vi "Connect Channel.vi"(7 "Channel Array in":refnum<class "CIFChannels.lvclass">[](array[class]), 8 "error in (no error)":errorcluster, 9 "Connection":T1 {"Custom Data" format="%.0x"}, 10 "Subscriber Name":string, 11 "CIFChannelMng in":refnum<class "CIFChannelMng.lvclass">) -> (0 "error out":errorcluster, 2 "Update OOB":bool, 3 "CIFChannelMng out":refnum<class "CIFChannelMng.lvclass">, 5 "Channel Array out":refnum<class "CIFChannels.lvclass">[](array[class]))   [LabVIEW 2021, in "CIFChannelMng.lvclass"]
uses:
  CIFChannelMng.lvclass
  CIFChannelMng.lvclass/CIFChannelMng.ctl
  <vilib>/CIF Foundation/CIF Channels Core/CIFChannels/Typedef/Channel State.ctl
  <vilib>/CIF Foundation/CIF Channels Core/CIFChannels/CIFChannels.lvclass
  <vilib>/CIF Foundation/CIF Channels Core/ChannelCommon/typedef/New FIFO Instance Response.ctl
  <vilib>/CIF Foundation/CIF Channels Core/ChannelCommon/ChannelCommon.lvlib
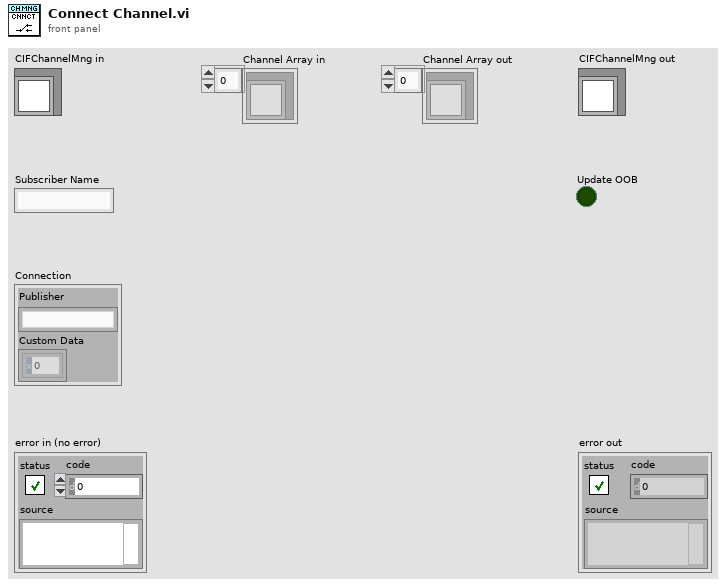
[diagram p1: front panel]
types:
  T1 = typedef "ChannelCommon.lvlib/New FIFO Instance Response.ctl" = cluster{"Publisher":string, "Custom Data":u8[]}
  T2 = typedef "CIFChannels.lvclass/Channel State.ctl" = enum16{"Creating", "Disconnected", "Connecting", "Connected", "Destroyed"}
  T3 = typedef "CIFChannelMng.lvclass/Channel List for OOB.ctl" = cluster{"Name":string, "Direction":T4, "Type":string, "Connected?":bool, "Connected Name":string, "Custom Config Data":u8[], "Forced?":bool, "Pattern":T5}
  T4 = typedef "CIFChannels.lvclass/Direction.ctl" = enum16{"Publisher", "Subscriber"}
  T5 = typedef "ChannelCommon.lvlib/Channel Pattern.ctl" = enum16{"Unknown", "Tag", "FIFO", "MultiFIFO", "BackpressureFIFO"}
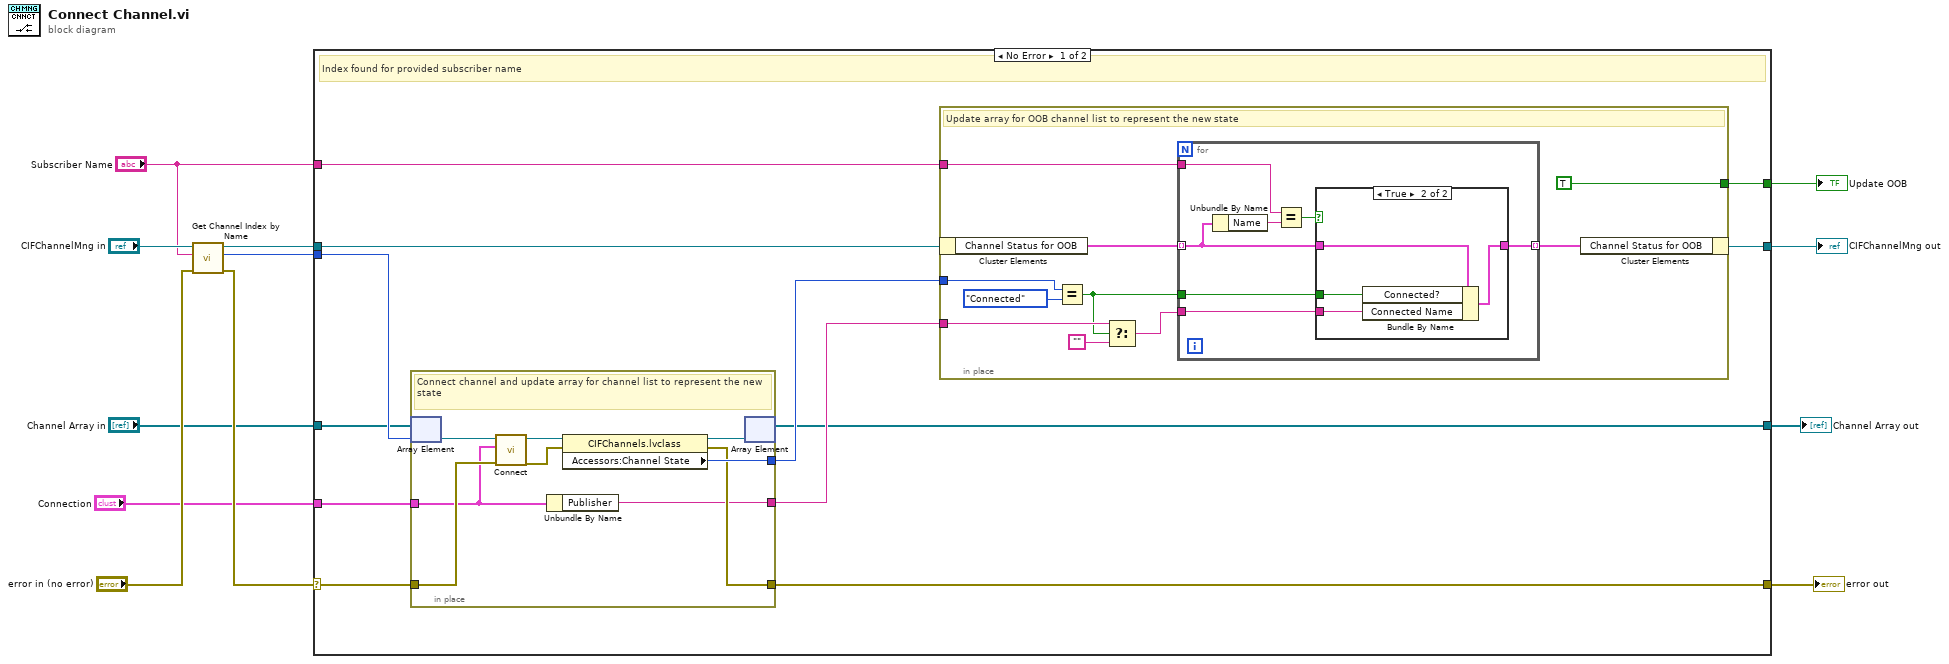
[diagram p0: block diagram]
diagram:
  n1 = call "Get Channel Index by Name.vi"("error in (no error)"="error in (no error)", "Channel Name"="Subscriber Name", "CIFChannelMng in"="CIFChannelMng in") -> ("error out"=w4:errorcluster, "Channel Index"=w5:i32, "CIFChannelMng out"=w6:refnum<class "CIFChannelMng.lvclass">)  [unwired: 6 in]
  n2 = case shown="No Error" w4 {
    selector: w4 -> [w23 w58]
    tunnel: w6 -> [w16 w57]
    tunnel: w5 -> [w24 _]
    tunnel: "Subscriber Name" -> [w20 _]
    tunnel: [w19 w57] -> w10
    tunnel: [w18 w58] -> w8
    tunnel: [w17 _] -> w7
    tunnel: "Channel Array in" -> [w15 w56]
    tunnel: [w14 w56] -> w2
    tunnel: "Connection" -> [w13 _]
    frame No Error {
      # "Index found for provided subscriber name"
      n3 = in-place {
        in-place-border: [w31] -> w22
        in-place-border: [w26] -> w21
        in-place-border: w23 -> [w29]
        in-place-border: [w27] -> w18
        in-place-border: w13 -> [w25]
        # "Connect channel and update array for channel list to represent the new state"
        n4 = in-place-array #1(w15, w24) -> (w30:refnum<class "CIFChannels.lvclass">)
        n5 = call-dynamic "Connect.vi"("error in (no error)"=w29, "Connection"=w25, "CIFChannels in"=w30) -> ("error out"=w32:errorcluster, "CIFChannels out"=w33:refnum<class "CIFChannels.lvclass">)  [unwired: 7 in]
        n6 = Unbundle By Name(w25) -> ("Publisher"=w26:string)
        n7 = property class="CIFChannels.lvclass"(reference=w33, error in=w32) -> (reference out=w28:refnum<class "CIFChannels.lvclass">, error out=w27:errorcluster, "Accessors:Channel State"=w31:T2)
        n8 = in-place-array #1(w28) -> (w14:refnum<class "CIFChannels.lvclass">[])  [unwired: 1 out]
      }
      n9 = in-place {
        in-place-border: w21 -> [w42]
        in-place-border: w22 -> [w38]
        in-place-border: w20 -> [w35]
        in-place-border: [TRUE ("Update OOB")] -> w17
        # "Update array for OOB channel list to represent the new state"
        n10 = in-place-cluster #2(w16) -> ("Channel Status for OOB"=w37:T3[])
        n11 = Equal?(x=w38, y=Channel_State."Connected") -> (x = y?=w40:bool)
        n12 = Select(t=w42, s=w40, f="") -> (s? t:f=w39:string)
        n13 = for {
          tunnel: w37 -> [w49] mode=indexing
          tunnel: w40 -> [w48]
          tunnel: w39 -> [w47]
          tunnel: [w46] -> w36 mode=indexing
          tunnel: w35 -> [w44]
          n14 = Unbundle By Name(w49) -> ("Name"=w50:string)
          n15 = Equal?(x=w44, y=w50) -> (x = y?=w45:bool)
          n16 = case shown="True" w45 {
            tunnel: w49 -> [w51 w55]
            tunnel: w48 -> [_ w54]
            tunnel: w47 -> [_ w53]
            tunnel: [w51 w52] -> w46
            frame False {
            }
            frame True {
              n17 = Bundle By Name(cluster=w55, "Connected?"=w54, "Connected Name"=w53) -> (w52:T3)
            }
          }
        }
        n18 = in-place-cluster #2("Channel Status for OOB"=w36) -> (w19:refnum<class "CIFChannelMng.lvclass">)
      }
    }
    frame Error {
      # "Index by name created error"
    }
  }
  "error out" <- w8
  "CIFChannelMng out" <- w10
  "Update OOB" <- w7
  "Channel Array out" <- w2
